vi "Configure Resistance.vi"(8 "error in (no error)":errorcluster, 9 "Resistance Integration Time (10: 10)":dbl(ring)=10.0 items=["0.02"=0.02, "0.2"=0.2, "1"=1.0, "10"=10.0, "100"=100.0], 10 "Resistance Type (0: Resistance 2-wire)":i32(ring) items=["Resistance 2-wire", "Resistance 4-wire"], 11 "VISA resource name":refnum<visa-resource-name>) -> (0 "error out":errorcluster, 3 "VISA resource name out":refnum<visa-resource-name>)   [LabVIEW 2013, in "Agilent 3446X Series.lvlib"]
doc: "Configures the settings for resistance measurements."
uses:
  Agilent 3446X Series.lvlib
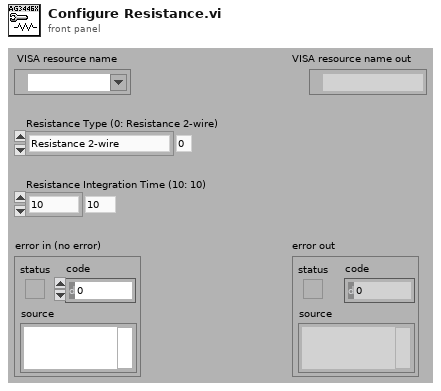
[diagram p1: front panel]
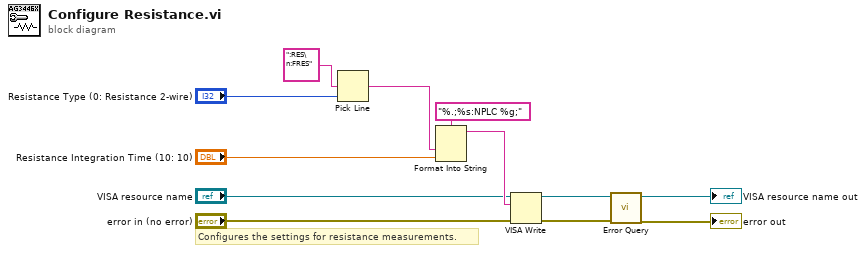
[diagram p0: block diagram]
diagram:
  # "Configures the settings for resistance measurements."
  n1 = Pick Line(multi-line string=":RES\n:FRES", line index="Resistance Type (0: Resistance 2-wire)") -> (output string=w9:string)  [unwired: 1 out]
  n2 = Format Into String(format string="%.;%s:NPLC %g;", w9, "Resistance Integration Time (10: 10)") -> (resulting string=w7:string)  [unwired: 2 in, 1 out]
  n3 = VISA Write(VISA resource name="VISA resource name", write buffer=w7, error in (no error)="error in (no error)") -> (VISA resource name out=w4:refnum<visa-resource-name>, error out=w3:errorcluster)  [unwired: 1 out]
  n4 = call "Error Query.vi"("error in (no error)"=w3, "VISA resource name"=w4) -> ("error out"=→"error out":errorcluster, "VISA resource name out"=→"VISA resource name out":refnum<visa-resource-name>)  [unwired: 8 out]
